vi "add_colorRGBA.vi"(6 "Color RBGA":cluster{"B":sgl, "R":i32, "G":i32, "A":dbl}={"B"=20.0, "R"=0, "G"=0, "A"=0.0}, 7 "msg in":string) -> (3 "msg out":string)   [LabVIEW 2012]
doc: "Flattens an color RGBA into a message"
uses:
  <userlib>/ROS for LabVIEW Software/ROS/MessageBuilding/std_msgs/subs/float32Scalar.vi
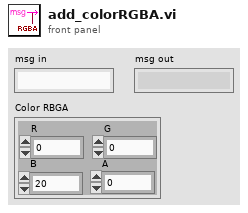
[diagram p1: front panel]
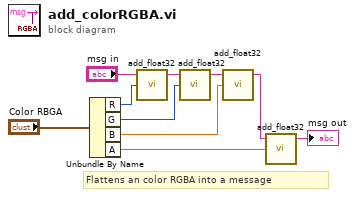
[diagram p0: block diagram]
diagram:
  # "Flattens an color RGBA into a message"
  n1 = Unbundle By Name("Color RBGA") -> ("R"=w8:i32, "G"=w5:i32, "B"=w6:sgl, "A"=w3:dbl)
  n2 = call-poly <userlib>:"add_float32.vi"("Numeric"=w8, "msg in"="msg in") -> ("msg out"=w7:string)  [unwired: 3 in]
  n3 = call-poly <userlib>:"add_float32.vi"("Numeric"=w5, "msg in"=w7) -> ("msg out"=w4:string)  [unwired: 3 in]
  n4 = call-poly <userlib>:"add_float32.vi"("Numeric"=w6, "msg in"=w4) -> ("msg out"=w2:string)  [unwired: 3 in]
  n5 = call-poly <userlib>:"add_float32.vi"("Numeric"=w3, "msg in"=w2) -> ("msg out"=→"msg out":string)  [unwired: 3 in]
